vi "TP 1.6 Sub VI.vi"(1 "Temp inicial":dbl) -> (0 "Numeric":dbl)   [LabVIEW 2013]
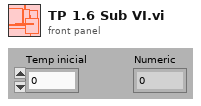
[diagram p1: front panel]
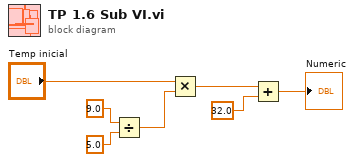
[diagram p0: block diagram]
diagram:
  n1 = Divide(x=9.0, y=5.0) -> (x/y=w3:dbl)
  n2 = Multiply(x="Temp inicial", y=w3) -> (x*y=w4:dbl)
  n3 = Add(x=w4, y=32.0) -> (x+y=→"Numeric":dbl)
